vi "SVT Gears.vi"(0 "number of gear1 teeth":u32=17 min=1, 1 "gear1 nominal speed [RPM]":dbl=1200.0, 2 "desired units":u16(ring) items=["Hz", "Order"], 5 "number of gear2 teeth":u32=53 min=1, 11 "error in (no error)":errorcluster) -> (3 "gear2 nominal speed [RPM]":dbl=384.9056603773585, 4 "gear mesh frequency":dbl=340.0, 6 "gear assembly phase frequency":dbl=340.0, 8 "hunting tooth frequency":dbl=0.37735849056603776, 15 "error out":errorcluster)   [LabVIEW 2017, in "SoundVib_MachineCharacteristic.lvlib"]
doc: "Calculates characteristic frequencies or orders of gearboxes."
uses:
  <vilib>/addons/Sound and Vibration/svt_Machine Characteristic/SoundVib_MachineCharacteristic.lvlib
  <vilib>/gmath/NI_Gmath.lvlib
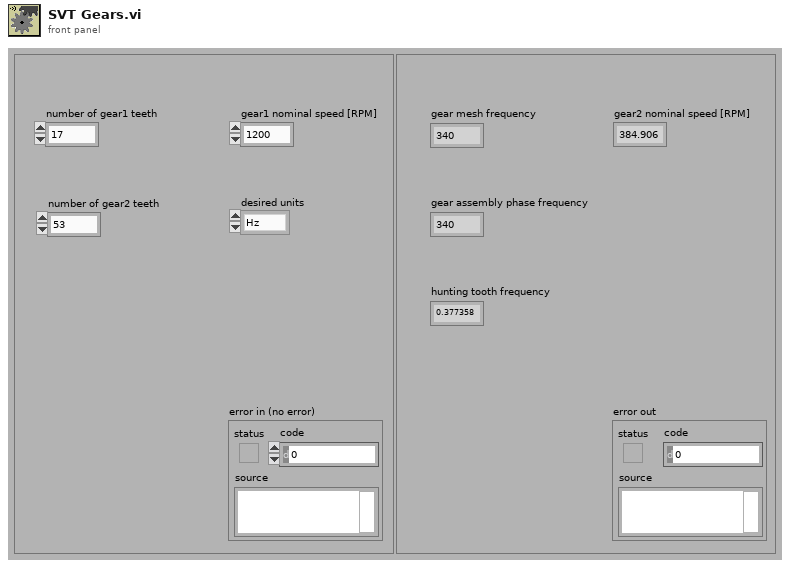
[diagram p1: front panel]
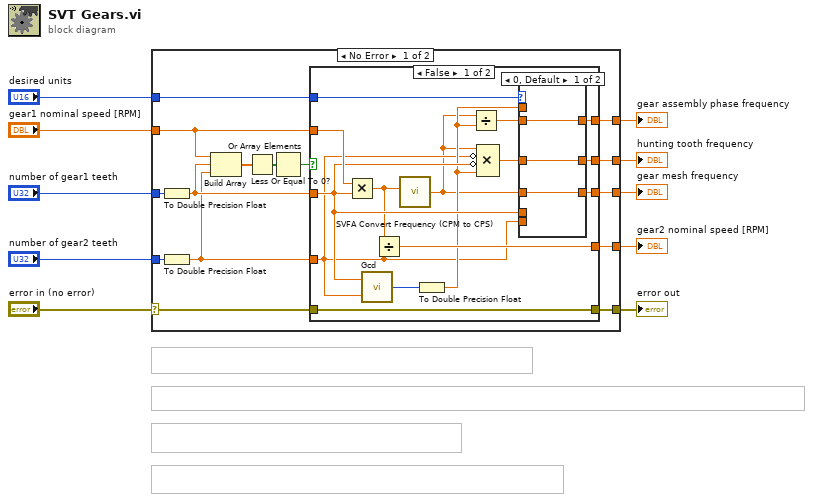
[diagram p0: block diagram]
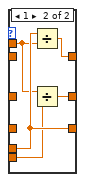
[diagram p2: hidden frame]
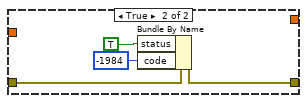
[diagram p3: hidden frame]
diagram:
  n1 = case shown="No Error" "error in (no error)" {
    selector: "error in (no error)" -> [w25 w53]
    tunnel: [w24 w53] -> w9
    tunnel: "gear1 nominal speed [RPM]" -> [w16 _]
    tunnel: "number of gear1 teeth" -> [w18 _]
    tunnel: "number of gear2 teeth" -> [w17 _]
    tunnel: [w23 _] -> w5
    tunnel: [w22 _] -> w4
    tunnel: [w21 _] -> w3
    tunnel: [w20 _] -> w2
    tunnel: "desired units" -> [w19 _]
    frame No Error {
      n2 = To Double Precision Float(number=w18) -> (double precision float=w15:dbl)
      n3 = To Double Precision Float(number=w17) -> (double precision float=w14:dbl)
      n4 = Build Array(w16, w15, w14) -> (w13:dbl[])
      n5 = Less Or Equal To 0?(x=w13) -> (x <= 0?=w12:bool[])
      n6 = Or Array Elements(Boolean array=w12) -> (logical OR=w11:bool)
      n7 = case shown="False" w11 {
        tunnel: w25 -> [w40 w52]
        tunnel: [w40 w51] -> w24
        tunnel: w16 -> [w32 _]
        tunnel: w14 -> [w28 _]
        tunnel: [w39 _] -> w23
        tunnel: [w37 _] -> w22
        tunnel: [w33 _] -> w21
        tunnel: [w35 _] -> w20
        tunnel: w19 -> [w38 _]
        tunnel: w15 -> [w30 _]
        frame False {
          n8 = Multiply(x=w32, y=w30) -> (x*y=w27:dbl)
          n9 = call <vilib>:"Gcd.vi"("y"=w28, "x"=w30) -> ("gcd(x,y)"=w31:i32)
          n10 = Divide(x=w27, y=w28) -> (x/y=w39:dbl)
          n11 = call <vilib>:"SVFA Convert Frequency (CPM to CPS).vi"("nominal speed [RPM]"=w27) -> ("frequency [Hz]"=w26:dbl)  [unwired: 5 in]
          n12 = To Double Precision Float(number=w31) -> (double precision float=w29:dbl)
          n13 = Divide(x=w26, y=w29) -> (x/y=w34:dbl)
          n14 = Compound Arithmetic op=MULTIPLY(w26, invert w28, invert w30, w29) -> (w36:dbl)
          n15 = case shown="0, Default" w38 {
            tunnel: w26 -> [w43 _]
            tunnel: [w43 w47] -> w37
            tunnel: w36 -> [w42 _]
            tunnel: [w42 w46] -> w35
            tunnel: [w41 w48] -> w33
            tunnel: w34 -> [w41 _]
            tunnel: w30 -> [_ w47]
            tunnel: w29 -> [_ w44]
            tunnel: w28 -> [_ w45]
            frame 0, Default {
            }
            frame 1 {
              n16 = Divide(x=w47, y=w44) -> (x/y=w48:dbl)
              n17 = Divide(x=w44, y=w45) -> (x/y=w46:dbl)
            }
          }
        }
        frame True {
          n18 = Bundle By Name(cluster=w52, "status"=TRUE, "code"=-1984) -> (w51:errorcluster)
        }
      }
    }
    frame Error {
    }
  }
  "gear2 nominal speed [RPM]" <- w5
  "gear mesh frequency" <- w4
  "gear assembly phase frequency" <- w3
  "hunting tooth frequency" <- w2
  "error out" <- w9
